vi "ConvertValveStateToDisplay.vi"(11 "Valve State":T2) -> (3 "MFC Valve State":T1)   [LabVIEW 2012]
uses:
  libs/Sierra-M100/Public/Controls/ValveState.ctl
  MFCDisplayValveState.ctl
  libs/Sierra-M100/Sierra-M100.lvlib
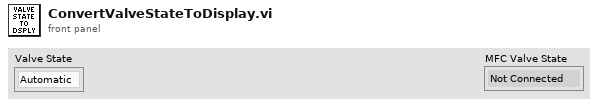
[diagram p1: front panel]
types:
  T1 = typedef "MFCDisplayValveState.ctl" = enum16{"Not Connected", "Automatic", "Closed", "Purge"}
  T2 = typedef "Sierra-M100.lvlib/ValveState.ctl" = enum16{"Automatic", "Closed", "Purge"}
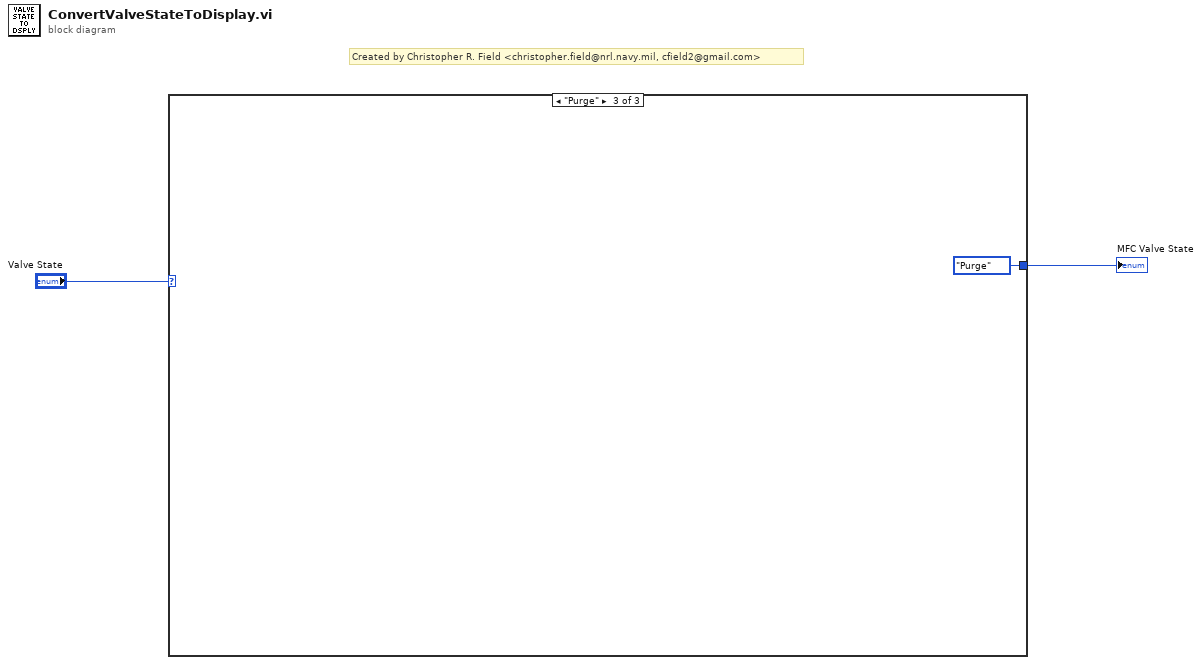
[diagram p0: block diagram]
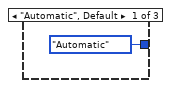
[diagram p2: hidden frame]
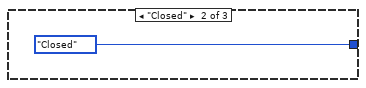
[diagram p3: hidden frame]
diagram:
  # "Created by Christopher R. Field <christopher.field@nrl.navy.mil, cfield2@gmail.com>"
  n1 = case shown="\"Purge\"" "Valve State" {
    tunnel: [MFCDisplayValveState."Automatic" ("MFC Valve State") MFCDisplayValveState."Closed" ("MFC Valve State") MFCDisplayValveState."Purge" ("MFC Valve State")] -> w1
    frame "Automatic", Default {
    }
    frame "Closed" {
    }
    frame "Purge" {
    }
  }
  "MFC Valve State" <- w1
